vi "GD_buider.vi"(7 "GD":bool, 11 "Event type":string="BCG") -> (3 "TACS / MODELS":string)   [LabVIEW 2020]
uses:
  <vilib>/Utility/file.llb/Read Delimited Spreadsheet (string).vi
panel:
  out "GDs nodes":string[](array[string])
  in  "Lista de condições (arquivo.txt) 2":string="GDs.txt"
  in  "Diretório de trabalho":path=path "C:/ATP/ATPDraw/Projects_Flavio"
  # "TACS / MODEL BUILDER PARA GD"
  # "GDs em ordem numérica., indepentente dos nós (ex. 1, 2, 3... etc)\n- Locais (nós) são definidos pela chave"
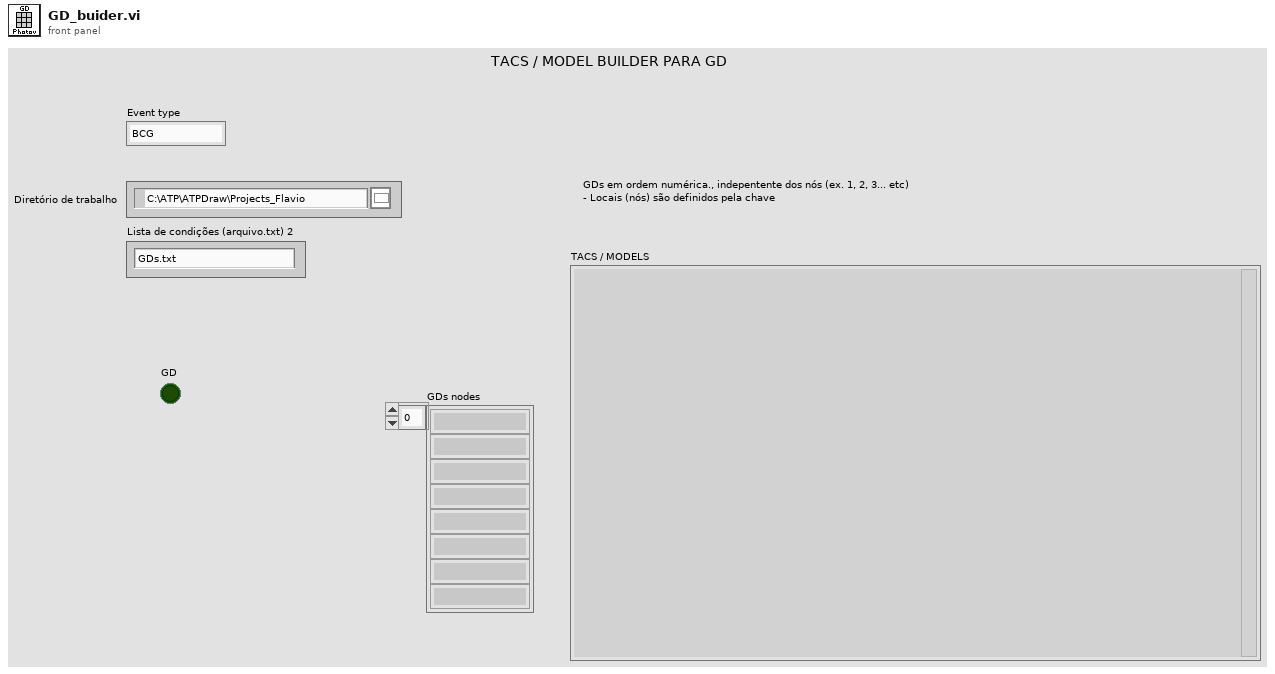
[diagram p1: front panel]
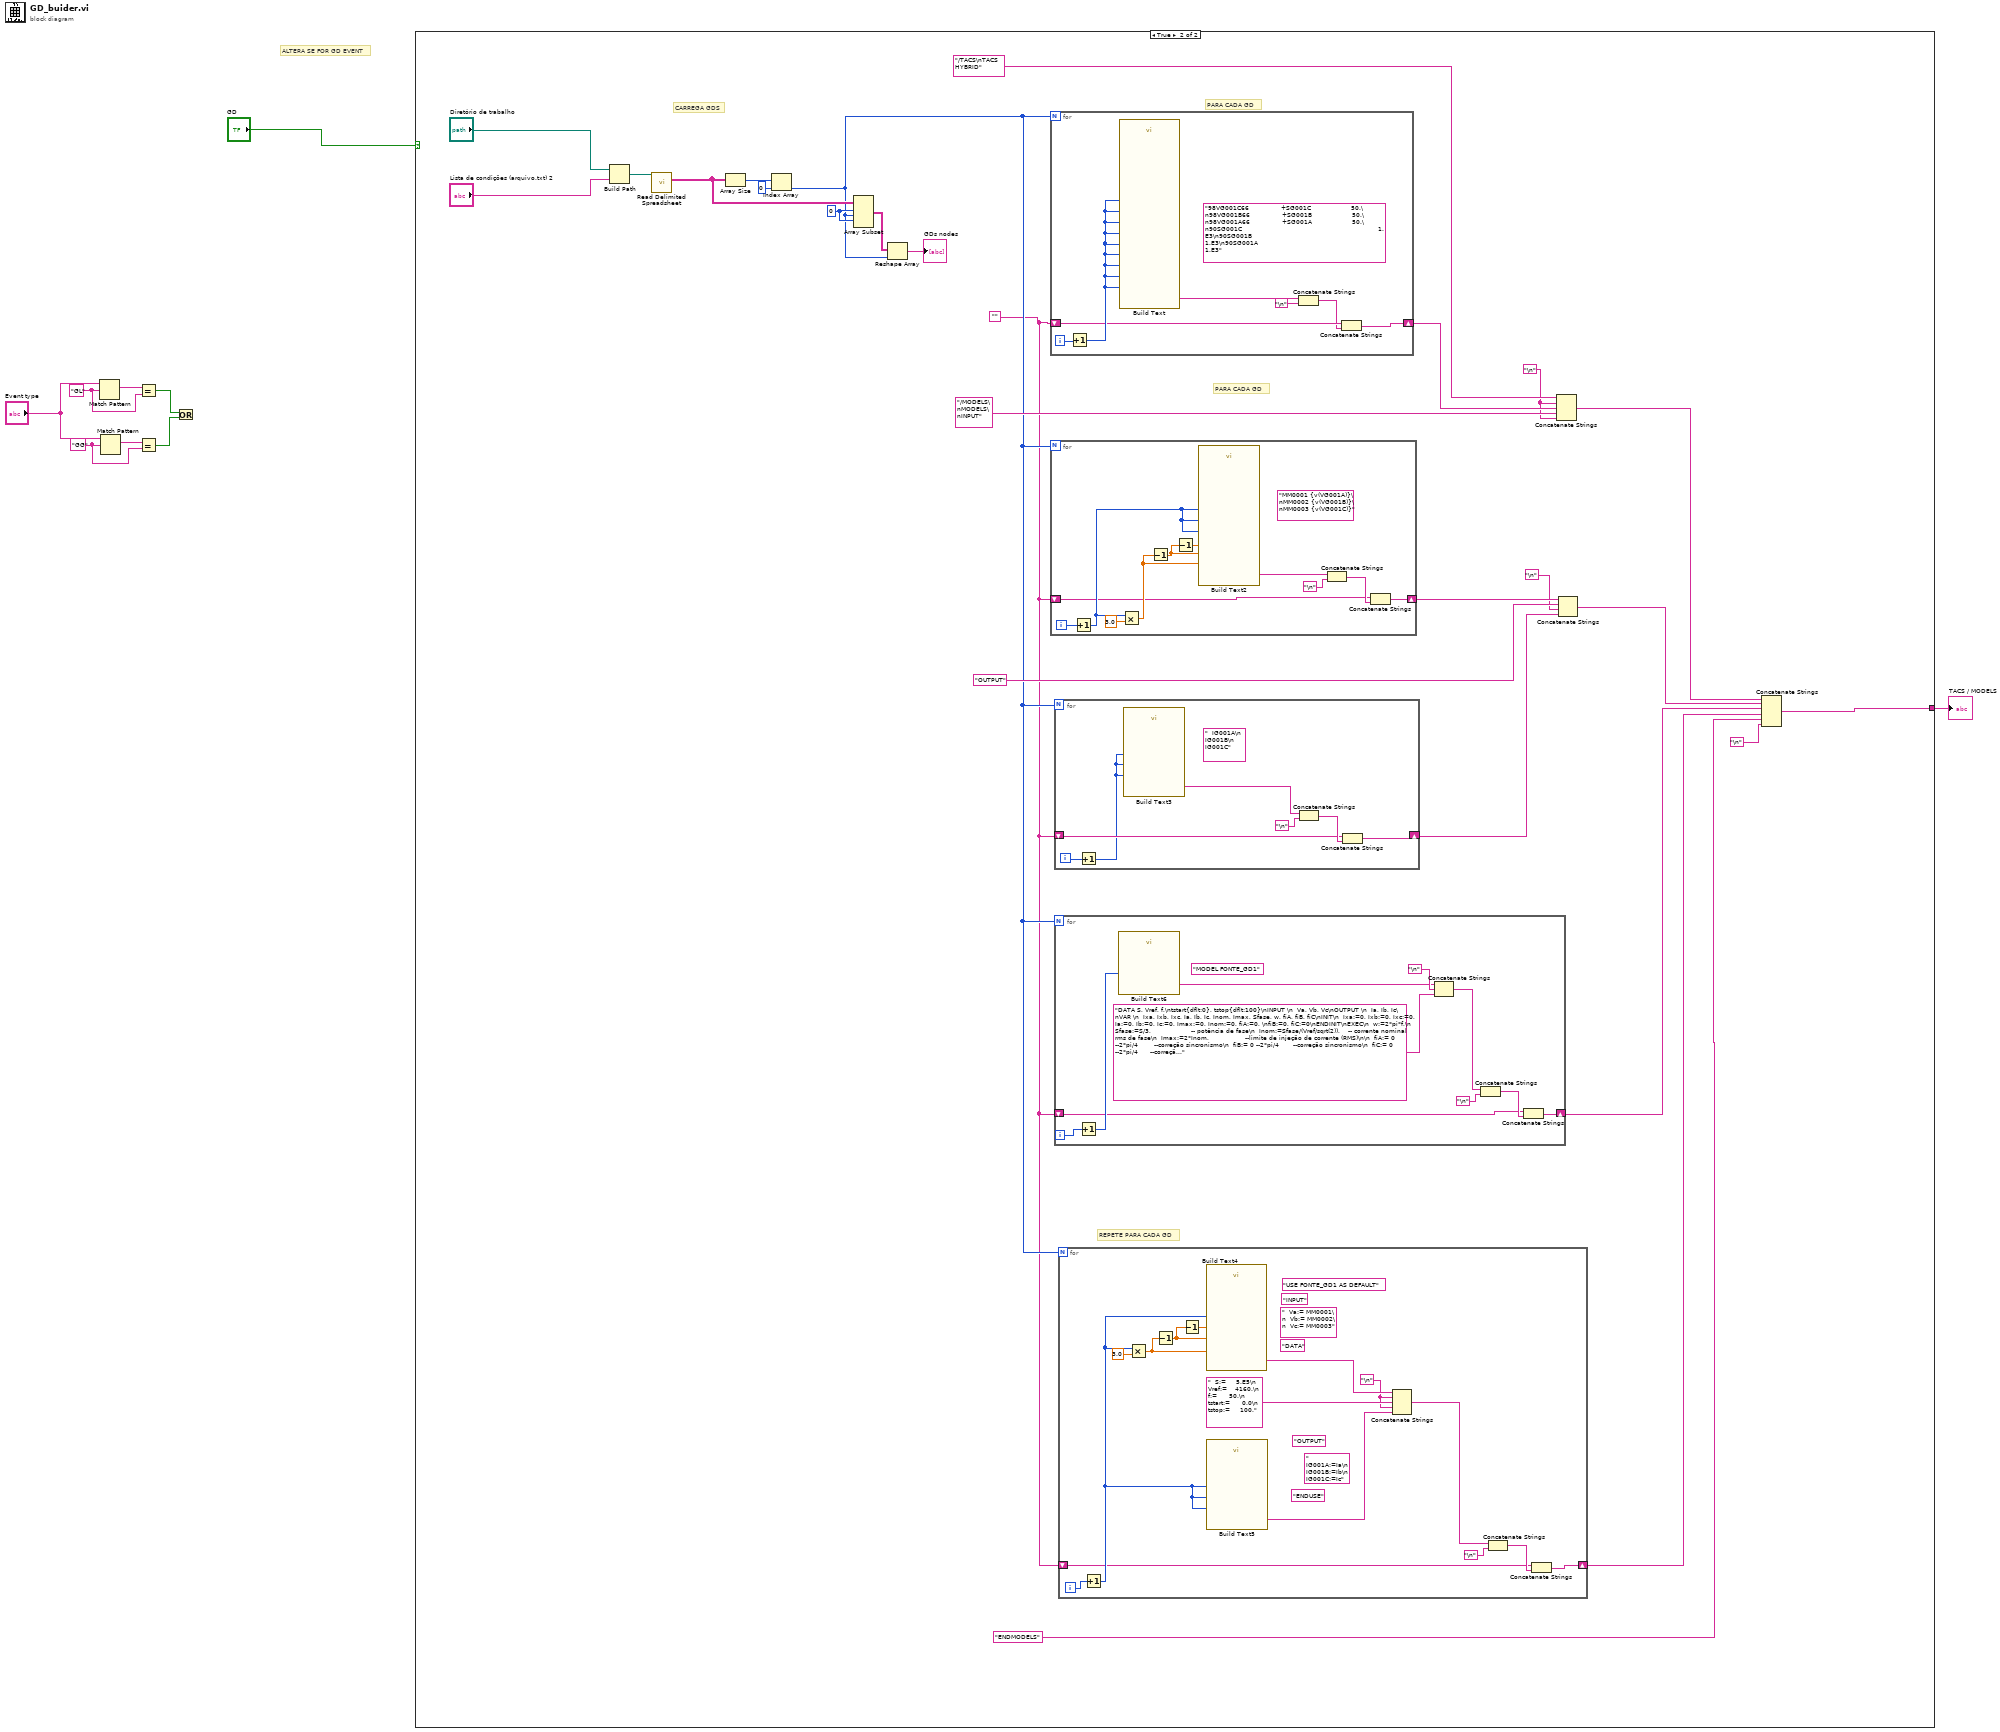
[diagram p0: block diagram]
diagram:
  w7 = "GL" ("regular expression")
  w5 = "GG" ("regular expression")
  # "ALTERA SE FOR GD EVENT"
  n1 = Match Pattern(string="Event type", regular expression=w7) -> (match substring=w6:string)  [unwired: 1 in, 3 out]
  n2 = Match Pattern(string="Event type", regular expression=w5) -> (match substring=w8:string)  [unwired: 1 in, 3 out]
  n3 = Equal?(x=w6, y=w7) -> (x = y?=w3:bool)
  n4 = Equal?(x=w8, y=w5) -> (x = y?=w4:bool)
  n5 = Or(x=w3, y=w4) -> ()  [unwired: 1 out]
  n6 = case shown="True" "GD" {
    tunnel: [_ w33] -> w9
    frame False {
    }
    frame True {
      w10 = ""
      w28 = 0 ("index")
      w17 = "\n"
      # "PARA CADA GD"
      # "CARREGA GDS"
      # "PARA CADA GD"
      # "REPETE PARA CADA GD"
      n7 = Build Path(base path="Diretório de trabalho", name or relative path="Lista de condições (arquivo.txt) 2") -> (appended path=w30:path)
      n8 = call-poly <vilib>:"Read Delimited Spreadsheet.vi"("file path (dialog if empty)"=w30) -> ("all rows"=w27:string[][])  [unwired: 9 in, 5 out]
      n9 = Array Size(array=w27) -> (size(s)=w26:i32[])
      n10 = Index Array(array=w26, index=0) -> (element=w18:i32)
      n11 = Array Subset(array=w27, index (row)=w28, length (row)=w18, index (col)=w28) -> (w24:string[][])  [unwired: 1 in]
      n12 = Reshape Array(w24, w18) -> (→"GDs nodes":string[])
      n13 = for {
        N: w18 -> [_]
        shift-right: [w79] -> w32
        shift-left: w10 -> [w81]
        i -> [w85]
        (unwired) "98VG001C66                +SG001C                    50.\n98VG001B66                +SG001B                    50.\n98VG001A66                +SG001A                    50.\n90SG001C                                                                    1.E3\n90SG001B                                                                    1.E3\n90SG001A                                                                    1.E3"
        n14 = Increment(x=w85) -> (x+1=w84:i32)
        n15 = call "Build Text"("vg_c"=w84, "sg_c2"=w84, "vg_b"=w84, "sg_b2"=w84, "vg_a"=w84, "sg_a2"=w84, "sg_c"=w84, "sg_b"=w84, "sg_a"=w84) -> ("Result"=w82:string)  [unwired: 17 in, 1 out]
        n16 = Concatenate Strings(w82, "\n") -> (w80:string)
        n17 = Concatenate Strings(w81, w80) -> (w79:string)
      }
      n18 = for {
        N: w18 -> [_]
        shift-right: [w70] -> w34
        shift-left: w10 -> [w69]
        i -> [w75]
        (unwired) "MM0001 {v(VG001A)}\nMM0002 {v(VG001B)}\nMM0003 {v(VG001C)}"
        n19 = Increment(x=w75) -> (x+1=w74:i32)
        n20 = Multiply(x=w74, y=3.0) -> (x*y=w73:dbl)
        n21 = Decrement(x=w73) -> (x-1=w77:dbl)
        n22 = Decrement(x=w77) -> (x-1=w78:dbl)
        n23 = call "Build Text2"("vg_b"=w74, "vg_c"=w74, "mm_a"=w78, "vg_a"=w74, "mm_b"=w77, "mm_c"=w73) -> ("Result"=w68:string)  [unwired: 8 in, 1 out]
        n24 = Concatenate Strings(w68, "\n") -> (w71:string)
        n25 = Concatenate Strings(w69, w71) -> (w70:string)
      }
      n26 = for {
        N: w18 -> [_]
        shift-right: [w65] -> w19
        shift-left: w10 -> [w64]
        i -> [w62]
        (unwired) "  IG001A\n  IG001B\n  IG001C"
        n27 = Increment(x=w62) -> (x+1=w61:i32)
        n28 = call "Build Text3"("ig_a"=w61, "ig_b"=w61, "ic_c"=w61) -> ("Result"=w63:string)  [unwired: 11 in, 1 out]
        n29 = Concatenate Strings(w63, "\n") -> (w66:string)
        n30 = Concatenate Strings(w64, w66) -> (w65:string)
      }
      n31 = for {
        N: w18 -> [_]
        shift-right: [w53] -> w15
        shift-left: w10 -> [w51]
        i -> [w60]
        (unwired) "MODEL FONTE_GD1"
        n32 = Increment(x=w60) -> (x+1=w59:i32)
        n33 = call "Build Text6"("gd"=w59) -> ("Result"=w57:string)  [unwired: 13 in, 1 out]
        n34 = Concatenate Strings(w57, "\n", "DATA S, Vref, f,\ntstart{dflt:0}, tstop{dflt:100}\nINPUT \n  Va, Vb, Vc\nOUTPUT \n  Ia, Ib, Ic\nVAR \n  Ixa, Ixb, Ixc, Ia, Ib, Ic, Inom, Imax, Sfase, w, fiA, fiB, fiC\nINIT\n  Ixa:=0, Ixb:=0, Ixc:=0, Ia:=0, Ib:=0, Ic:=0, Imax:=0, Inom:=0, fiA:=0, \nfiB:=0, fiC:=0\nENDINIT\nEXEC\n  w:=2*pi*f,\n  Sfase:=S/3,                    -- potência de fase\n  Inom:=Sfase/(Vref/sqrt(2)),    -- corrente nominal rms de fase\n  Imax:=2*Inom,                  --limite de injeção de corrente (RMS)\n\n  fiA:= 0 --2*pi/4        --correção sincronismo\n  fiB:= 0 --2*pi/4       --correção sincronismo\n  fiC:= 0 --2*pi/4      --correção sincronismO\n----------------------------------------------------------------------\n\nIF t>tstart and t<0.02 THEN    --tempo em que ocorre a medida do valor rms a partir do inicio da simulação\n    Ia:=(Inom*(cos(w*t +fiA)))*sqrt(2)        \n    Ib:=(Inom*(cos(w*t-2*pi/3 +fiB)))*sqrt(2)        \n    Ic:=(Inom*(cos(w*t+2*pi/3 +fiC)))*sqrt(2)   \nENDIF\n\n---------------------------------------------------------------------\nIF t>0.02 and t<tstop THEN\n  \n  IF Va=0 THEN   \n    Ixa:=(Imax*(cos(w*t +fiA)))*sqrt(2)             \n  ELSE\n    Ixa:=(Sfase/Va)*(cos(w*t +fiA))*sqrt(2)  \n    IF abs(Ixa) > 2*(Inom*sqrt(2))THEN\n       Ixa:=(Imax*(cos(w*t +fiA)))*sqrt(2) \n    ENDIF\n  ENDIF\nIa:=Ixa\n\n  IF Vb=0 THEN   \n    Ixb:=(Imax*(cos(w*t-2*pi/3 +fiB)))*sqrt(2)     \n  ELSE\n    Ixb:=(Sfase/Vb)*(cos(w*t-2*pi/3 +fiB))*sqrt(2)  \n    IF abs(Ixb) > 2*(Inom*sqrt(2)) THEN\n       Ixb:=(Imax*(cos(w*t-2*pi/3 +fiB)))*sqrt(2)\n    ENDIF\n  ENDIF\nIb:=Ixb\n\n  IF Vc=0 THEN   \n    Ixc:=(Imax*(sin(w*t+2*pi/3 +fiC)))*sqrt(2)       \n  ELSE\n    Ixc:=(Sfase/Vc)*(cos(w*t+2*pi/3 +fiC))*sqrt(2)   \n    IF abs(Ixc) > 2*(Inom*sqrt(2)) THEN\n       Ixc:=(Imax*(cos(w*t+2*pi/3 +fiC)))*sqrt(2)\n    ENDIF\n  ENDIF\nIc:=Ixc\n\nENDIF\nENDEXEC\nENDMODEL") -> (w52:string)
        n35 = Concatenate Strings(w52, "\n") -> (w54:string)
        n36 = Concatenate Strings(w51, w54) -> (w53:string)
      }
      n37 = for {
        N: w18 -> [_]
        shift-right: [w38] -> w14
        shift-left: w10 -> [w37]
        i -> [w42]
        w43 = "\n"
        (unwired) "ENDUSE"
        (unwired) "  IG001A:=Ia\n  IG001B:=Ib\n  IG001C:=Ic"
        (unwired) "OUTPUT"
        (unwired) "DATA"
        (unwired) "  Va:= MM0001\n  Vb:= MM0002\n  Vc:= MM0003"
        (unwired) "INPUT"
        (unwired) "USE FONTE_GD1 AS DEFAULT"
        n38 = Increment(x=w42) -> (x+1=w41:i32)
        n39 = Multiply(x=w41, y=3.0) -> (x*y=w49:dbl)
        n40 = Decrement(x=w49) -> (x-1=w47:dbl)
        n41 = Decrement(x=w47) -> (x-1=w48:dbl)
        n42 = call "Build Text4"("mm_c"=w49, "gd"=w41, "mm_a"=w48, "mm_b"=w47) -> ("Result"=w46:string)  [unwired: 10 in, 1 out]
        n43 = call "Build Text5"("gd_a"=w41, "gd_b"=w41, "gd_c"=w41) -> ("Result"=w44:string)  [unwired: 11 in, 1 out]
        n44 = Concatenate Strings(w46, w43, "  S:=     5.E5\n  Vref:=    4160.\n  f:=      50.\n  tstart:=      0.0\n  tstop:=     100.", w43, w44) -> (w36:string)
        n45 = Concatenate Strings(w36, "\n") -> (w39:string)
        n46 = Concatenate Strings(w37, w39) -> (w38:string)
      }
      n47 = Concatenate Strings("/TACS\nTACS HYBRID", w17, w32, "/MODELS\nMODELS\nINPUT", w17) -> (w31:string)
      n48 = Concatenate Strings(w34, "OUTPUT", "\n", w19) -> (w16:string)
      n49 = Concatenate Strings(w31, w16, w15, w14, "ENDMODELS", "\n") -> (w33:string)
    }
  }
  "TACS / MODELS" <- w9
